vi "Initialize.vi"(8 "error in (no error)":errorcluster, 11 "State in":T1={"State"=enum."Idle", "Start Time"=timestamp(0 s since 1904-01-01), "Configuration"={"Cycle Period"=0.0, "Mettler"={"VISA resource name"="", "Simulated?"=FALSE}, "Scale Type"=""}, "Current Time"=timestamp(0 s since 1904-01-01), "First Iteration"=FALSE, "Data"={"Scale Read(g)"=0.0}, "Process Name"="", "Log Started"=FALSE}) -> (0 "error out":errorcluster, 3 "State out":T1={"State"=enum."Idle", "Start Time"=timestamp(0 s since 1904-01-01), "Configuration"={"Cycle Period"=0.0, "Mettler"={"VISA resource name"="", "Simulated?"=FALSE}, "Scale Type"=""}, "Current Time"=timestamp(0 s since 1904-01-01), "First Iteration"=FALSE, "Data"={"Scale Read(g)"=0.0}, "Process Name"="", "Log Started"=FALSE})   [LabVIEW 2018, in "Scale Module.lvlib" / "Scale Module Engine.lvlib"]
uses:
  Scale Module Engine.lvlib
  State Cluster.ctl
  State Enum.ctl
  Feed Module/Controls/Scale Module Settings Cluster.ctl
  Mettler Toledo/Controls/Settings Cluster.ctl
  Tag VIs/Tag FGV Operation Enum.ctl
  Mettler Toledo/Mettler Toledo.lvlib
  Shared Variables/Dynamic Shared Variables.lvlib
  Scale Module.lvlib
panel:
  # "Scale Settings"
  # "Scale Settings"
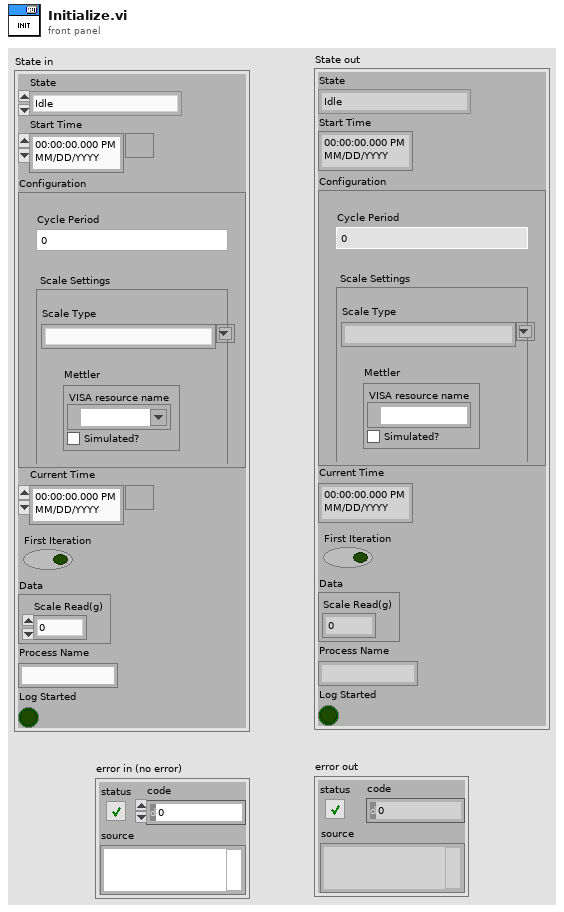
[diagram p1: front panel]
types:
  T1 = typedef "Scale Module.lvlib/Scale Module Engine.lvlib/State Cluster.ctl" = cluster{"State":T2, "Start Time":timestamp, "Configuration":T3, "Current Time":timestamp, "First Iteration":bool, "Data":cluster{"Scale Read(g)":dbl}, "Process Name":string, "Log Started":bool}
  T2 = typedef "Scale Module.lvlib/Scale Module Engine.lvlib/State Enum.ctl" = enum16{"Measuring", "Idle"}
  T3 = typedef "Scale Module.lvlib/Scale Module Settings Cluster.ctl" = cluster{"Cycle Period":dbl, "Mettler":T4, "Scale Type":string}
  T4 = typedef "Mettler Toledo.lvlib/Settings Cluster.ctl" = cluster{"VISA resource name":refnum<visa-resource-name>, "Simulated?":bool}
  T5 = typedef "Tag FGV Operation Enum.ctl" = enum16{"Init", "Set Notification Queue", "Create Tag", "Commit", "Write Tag (Numeric)", "Write Tag (Boolean)", "Read All Tags", "Read One Tag", "Delete Tag Category", "Set Alarm Parameters (Numeric)", "Set Alarm Parameters (Boolean)", "Enable All Alarms", "Disable All Alarms", "Delete All Tags", "Read Alarms", "Ack Alarm"}
  T6 = cluster{"Scale Tag":string, "Output Device Tag":string}
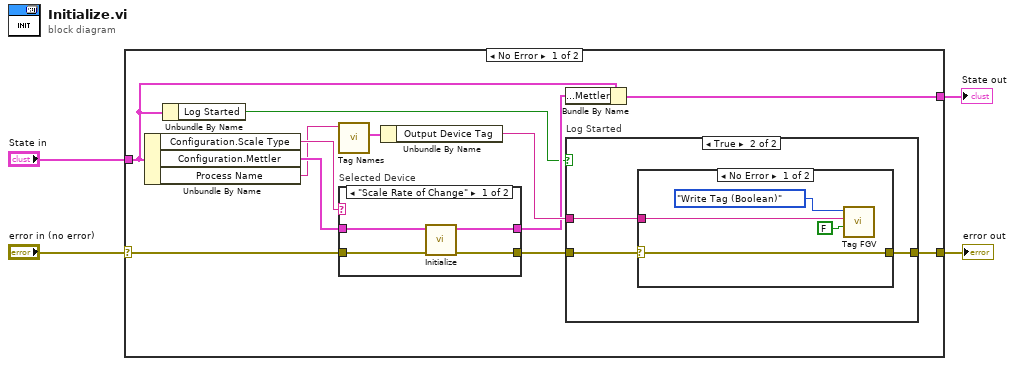
[diagram p0: block diagram]
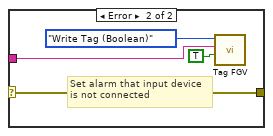
[diagram p3: hidden frame]
diagram:
  n1 = case shown="No Error" "error in (no error)" {
    selector: "error in (no error)" -> [w14 w36]
    tunnel: [w10 w36] -> w3
    tunnel: "State in" -> [w6 w35]
    tunnel: [w13 w35] -> w1
    frame No Error {
      n2 = Unbundle By Name(w6) -> ("Configuration.Scale Type"=w16:string, "Configuration.Mettler"=w15:T4, "Process Name"=w12:string)
      n3 = Unbundle By Name(w6) -> ("Log Started"=w5:bool)
      n4 = call "Tag Names.vi"("Process Name"=w12) -> ("Scale Tags"=w9:T6)  [unwired: 8 in, 2 out]
      n5 = case "Selected Device" shown="\"Scale Rate of Change\"" w16 {
        tunnel: w15 -> [w30 w34]
        tunnel: w14 -> [w29 w33]
        tunnel: [w31 w33] -> w11
        tunnel: [w32 w34] -> w7
        frame "Scale Rate of Change" {
          n6 = call "Initialize.vi"("error in (no error)"=w29, "Mettler Settings in"=w30) -> ("error out"=w31:errorcluster, "Mettler Settings out"=w32:T4)  [unwired: 7 in, 1 out]
        }
        frame "Default", Default {
        }
      }
      n7 = Unbundle By Name(w9) -> ("Output Device Tag"=w8:string)
      n8 = Bundle By Name(cluster=w6, "Configuration.Mettler"=w7) -> (w13:T1)
      n9 = case "Log Started" shown="True" w5 {
        tunnel: w11 -> [w17 w20]
        tunnel: [w17 w19] -> w10
        tunnel: w8 -> [_ w18]
        frame False {
        }
        frame True {
          n10 = case shown="No Error" w20 {
            selector: w20 -> [w24 w26]
            tunnel: [w24 w26] -> w19
            tunnel: w18 -> [w22 w25]
            frame No Error {
              n11 = call "Tag FGV.vi"("Data"=FALSE, "Tag Name"=w22, "Operation"=Tag_FGV_Operation_Enum."Write Tag (Boolean)") -> ()  [unwired: 3 in, 6 out]
            }
            frame Error {
              # "Set alarm that input device\nis not connected"
              n12 = call "Tag FGV.vi"("Data"=TRUE, "Tag Name"=w25, "Operation"=Tag_FGV_Operation_Enum."Write Tag (Boolean)") -> ()  [unwired: 3 in, 6 out]
            }
          }
        }
      }
    }
    frame Error {
    }
  }
  "error out" <- w3
  "State out" <- w1
